vi "获取周一日期.vi"() -> (2 "周一日期":string, 3 "FROM:":string)   [LabVIEW 2014]
panel:
  in  "日期格式":string="/"
  out "星期":string
  out "日":string
  out "月":string
  out "年":string
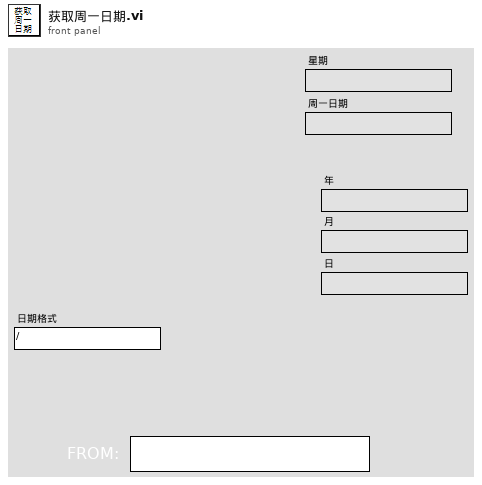
[diagram p1: front panel]
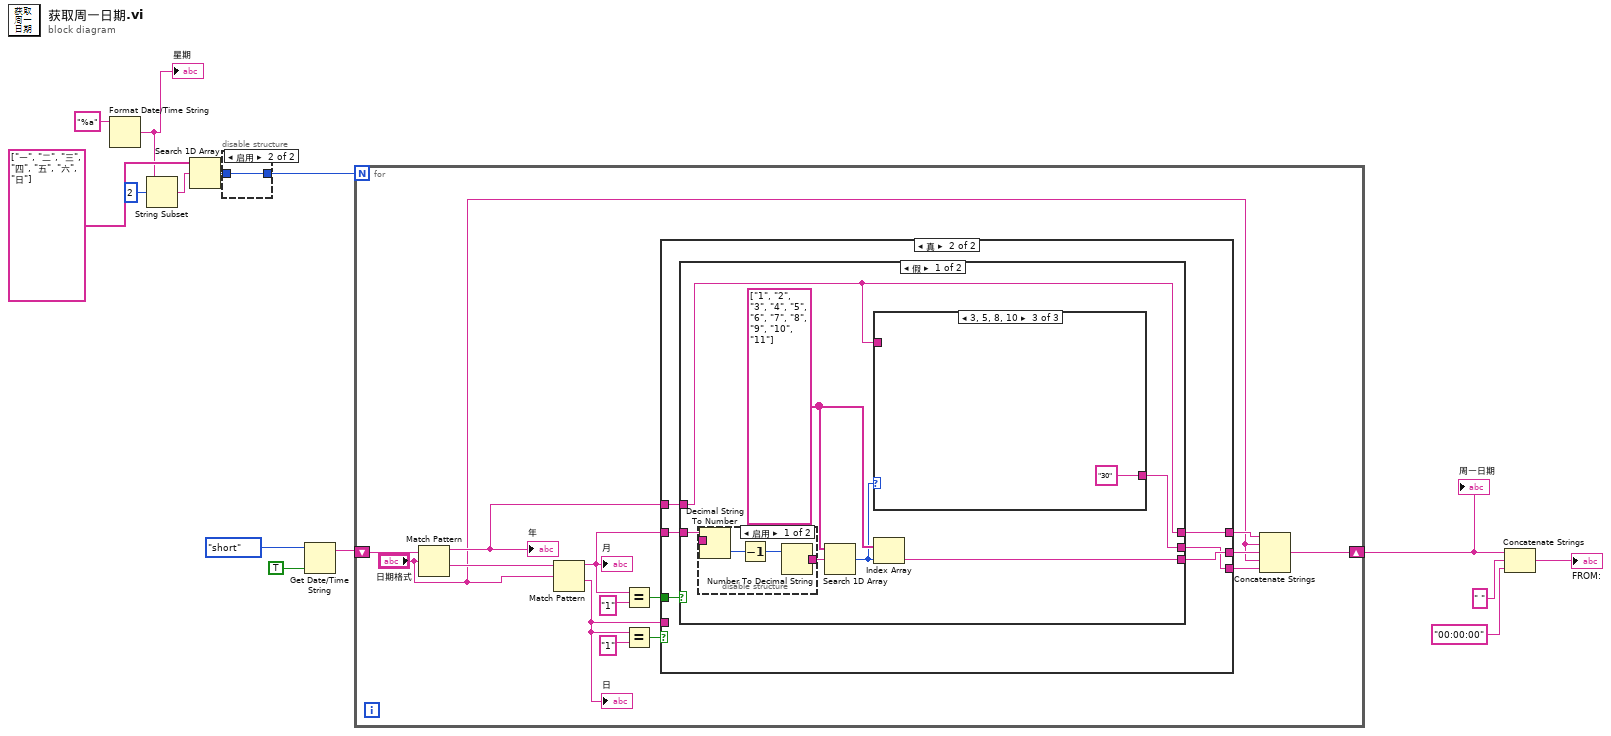
[diagram p0: block diagram]
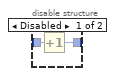
[diagram p2: hidden frame]
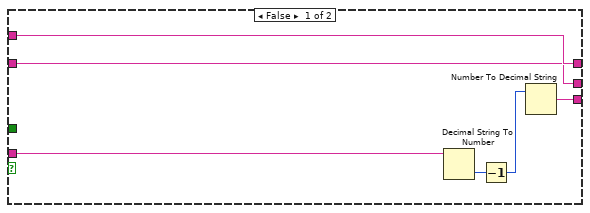
[diagram p3: hidden frame]
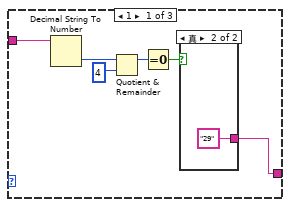
[diagram p5: hidden frame]
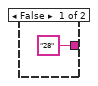
[diagram p6: hidden frame]
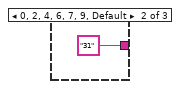
[diagram p7: hidden frame]
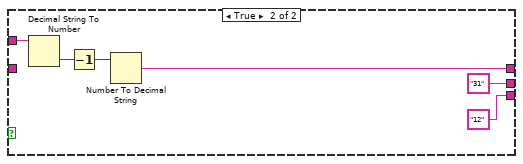
[diagram p8: hidden frame]
diagram:
  n1 = Format Date/Time String(time format string (%c)="%a" ("时间格式字符串(%c)")) -> (date/time string=w3:string)  [unwired: 2 in]
  "星期" <- w3
  n2 = String Subset(string=w3, offset (0)=2 ("偏移量(0)")) -> (substring=w2:string)  [unwired: 1 in]
  n3 = Search 1D Array(1D array=string[] ["一", "二", "三", "四", "五", "六", "日"] ("一维数组"), element=w2) -> (index of element=w6:i32)  [unwired: 1 in]
  n4 = disable-structure shown="启用" {
    disable-tunnel: w6 -> [w16 w17]
    disable-tunnel: [w15 w17] -> w4
    frame Disabled {
      n5 = Increment(x=w16) -> (x+1=w15:i32)
    }
    frame Enabled {
    }
  }
  n6 = Get Date/Time String(date format (0)=enum16{"short", "long", "abbreviated"}."short" ("日期格式(0)"), want seconds? (F)=TRUE ("需要秒？(F)")) -> (date string=w5:string)  [unwired: 1 in, 1 out]
  n7 = for {
    N: w4 -> [_]
    shift-right: [w23] -> w10
    shift-left: w5 -> [w20]
    n8 = Match Pattern(string=w20, regular expression="日期格式") -> (before substring=w22:string, after substring=w21:string)  [unwired: 1 in, 2 out]
    "年" <- w22
    n9 = Match Pattern(string=w21, regular expression="日期格式") -> (before substring=w25:string, after substring=w24:string)  [unwired: 1 in, 2 out]
    "月" <- w25
    "日" <- w24
    n10 = Equal?(x=w25, y="1") -> (x = y?=w28:bool)
    n11 = Equal?(x=w24, y="1") -> (x = y?=w29:bool)
    n12 = case shown="真" w29 {
      tunnel: w28 -> [_ w43]
      tunnel: w22 -> [w33 w42]
      tunnel: [w33 w41] -> w27
      tunnel: [w32 w40] -> w26
      tunnel: [w34 w39] -> w19
      tunnel: w25 -> [w32 w38]
      tunnel: w24 -> [w35 _]
      frame False {
        n13 = Decimal String To Number(string=w35) -> (number=w37:i32)  [unwired: 2 in, 1 out]
        n14 = Decrement(x=w37) -> (x-1=w36:i32)
        n15 = Number To Decimal String(number=w36) -> (decimal integer string=w34:string)  [unwired: 1 in]
      }
      frame True {
        n16 = case shown="假" w43 {
          tunnel: w42 -> [w46 w70]
          tunnel: [w46 w68] -> w41
          tunnel: [w47 "12" ("正则表达式")] -> w40
          tunnel: [w50 "31" ("正则表达式")] -> w39
          tunnel: w38 -> [w45 _]
          frame False {
            w49 = string[] ["1", "2", "3", "4", "5", "6", "7", "8", "9", "10", "11"] ("一维数组")
            n17 = disable-structure shown="启用" {
              disable-tunnel: w45 -> [w52 w55]
              disable-tunnel: [w51 w55] -> w44
              frame Enabled {
                n18 = Decimal String To Number(string=w52) -> (number=w53:i32)  [unwired: 2 in, 1 out]
                n19 = Decrement(x=w53) -> (x-1=w54:i32)
                n20 = Number To Decimal String(number=w54) -> (decimal integer string=w51:string)  [unwired: 1 in]
              }
              frame Disabled {
              }
            }
            n21 = Search 1D Array(1D array=w49, element=w44) -> (index of element=w48:i32)  [unwired: 1 in]
            n22 = case shown="3, 5, 8, 10" w48 {
              tunnel: [w56 "31" "30"] -> w50
              tunnel: w46 -> [w57 _ _]
              frame 1 {
                n23 = Decimal String To Number(string=w57) -> (number=w58:i32)  [unwired: 2 in, 1 out]
                n24 = Quotient & Remainder(x=w58, y=4) -> (x-y*floor(x/y)=w60:i32)  [unwired: 1 out]
                n25 = Equal To 0?(x=w60) -> (x = 0?=w61:bool)
                n26 = case shown="真" w61 {
                  tunnel: ["28" "29"] -> w56
                  frame False {
                  }
                  frame True {
                  }
                }
              }
              frame 0, 2, 4, 6, 7, 9, Default {
              }
              frame 3, 5, 8, 10 {
              }
            }
            n27 = Index Array(array=w49, index=w48) -> (element=w47:string)
          }
          frame True {
            n28 = Decimal String To Number(string=w70) -> (number=w69:i32)  [unwired: 2 in, 1 out]
            n29 = Decrement(x=w69) -> (x-1=w71:i32)
            n30 = Number To Decimal String(number=w71) -> (decimal integer string=w68:string)  [unwired: 1 in]
          }
        }
      }
    }
    n31 = Concatenate Strings(w27, "日期格式", w26, "日期格式", w19) -> (w23:string)
  }
  "周一日期" <- w10
  n32 = Concatenate Strings(w10, " " ("字符串"), "00:00:00" ("字符串")) -> (→"FROM:":string)
